vi "Read Pinch Strenght.vi"(6 "Multi-pinch":bool, 8 "Error In":errorcluster, 11 "Leap Handle In":T1) -> (0 "Error Out":errorcluster, 1 "Finger pinch":bool[](array[boolean]), 2 "Pinch Strength":sgl, 3 "Leap Handle Out":T1)   [LabVIEW 2014]
doc: "<b>Leap Read</b> requests and parses a <b>Frame</b> of data from the Leap Motion Controller. All the data associated with the Frame is organized into a LabVIEW cluster for accessibility.\n\nSpecifics about the data in the Frame cluster can be found by going to <b>Help » Leap Motion Controller Help</b> inside of LabVIEW"
uses:
  Typedef 2.0/Leap Handle.ctl
  C:/Users/Arquilla/Desktop/Smart Wristband/Leap Motion VIs 2.0/LeapCSharp.NET4.0.dll
  LeapCSharp.NET4.0.dll
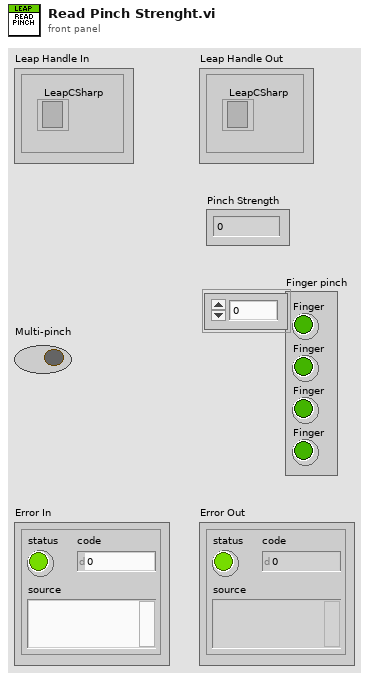
[diagram p1: front panel]
types:
  T1 = typedef "Leap Handle.ctl" = cluster{"LeapCSharp":refnum<k24>}
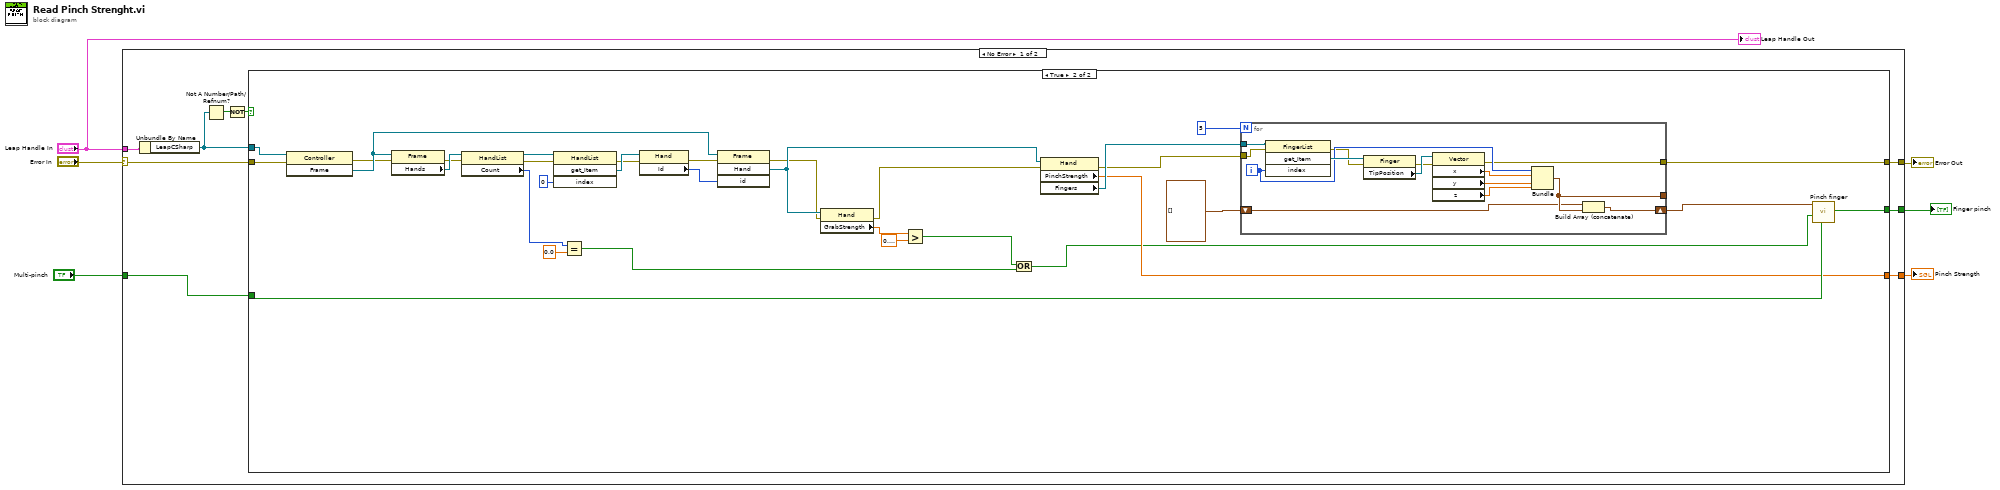
[diagram p0: block diagram]
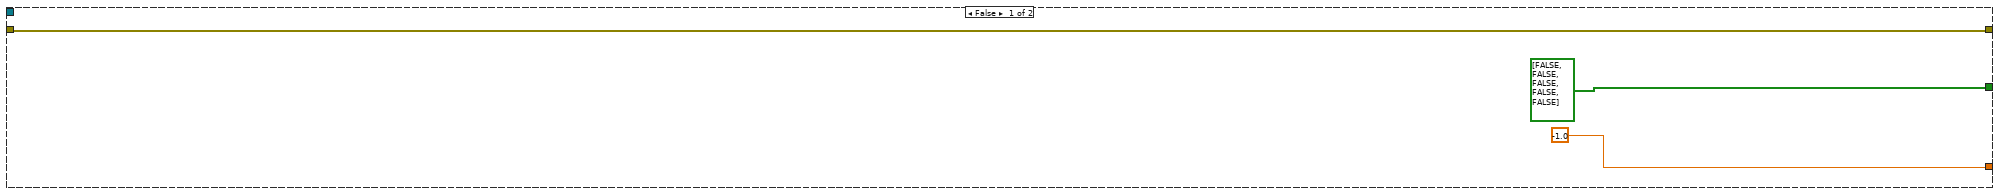
[diagram p2: hidden frame]
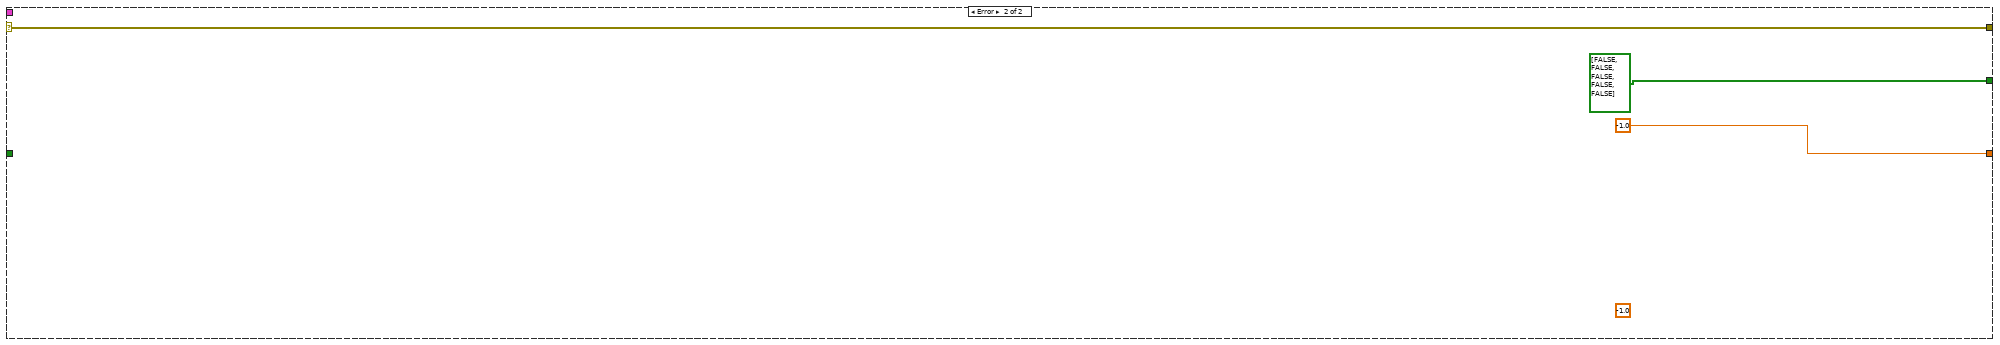
[diagram p3: hidden frame]
diagram:
  n1 = case shown="No Error" "Error In" {
    selector: "Error In" -> [w14 w67]
    tunnel: "Leap Handle In" -> [w15 _]
    tunnel: [w13 w67] -> w5
    tunnel: [w9 sgl -1.0 ("PinchStrength")] -> w3
    tunnel: [w8 bool[] [FALSE, FALSE, FALSE, FALSE, FALSE] ("Finger pinch")] -> w2
    tunnel: "Multi-pinch" -> [w7 _]
    frame No Error {
      n2 = Unbundle By Name(w15) -> ("LeapCSharp"=w10:refnum<k24>)
      n3 = Not A Number/Path/Refnum?(number/path/refnum=w10) -> (NaN/Path/Refnum?=w12:bool)
      n4 = Not(x=w12) -> (.not. x?=w11:bool)
      n5 = case shown="True" w11 {
        tunnel: w14 -> [w18 w38]
        tunnel: [w18 w36] -> w13
        tunnel: w10 -> [_ w39]
        tunnel: [sgl -1.0 ("GrabStrength") w24] -> w9
        tunnel: [bool[] [FALSE, FALSE, FALSE, FALSE, FALSE] ("Finger pinch") w37] -> w8
        tunnel: w7 -> [_ w35]
        frame False {
        }
        frame True {
          n6 = invoke class="Controller" method="Frame"(reference=w39, error in=w38) -> (error out=w44:errorcluster, "Frame"=w45:refnum<k24>)  [unwired: 1 in, 1 out]
          n7 = property class="Frame"(reference=w45, error in=w44) -> (error out=w43:errorcluster, "Hands"=w50:refnum<k24>)  [unwired: 1 out]
          n8 = property class="HandList"(reference=w50, error in=w43) -> (reference out=w49:refnum<k24>, error out=w42:errorcluster, "Count"=w22:i32)
          n9 = invoke class="HandList" method="get_Item"(reference=w49, error in=w42, "index"=0) -> (error out=w41:errorcluster, "get_Item"=w47:refnum<k24>)  [unwired: 1 in, 2 out]
          n10 = Equal?(x=w22, y=0.0) -> (x = y?=w20:bool)
          n11 = property class="Hand"(reference=w47, error in=w41) -> (error out=w40:errorcluster, "Id"=w46:i32)  [unwired: 1 out]
          n12 = invoke class="Frame" method="Hand"(reference=w45, error in=w40, "id"=w46) -> (error out=w27:errorcluster, "Hand"=w29:refnum<k24>)  [unwired: 1 in, 2 out]
          n13 = property class="Hand"(reference=w29, error in=w27) -> (error out=w26:errorcluster, "GrabStrength"=w28:sgl)  [unwired: 1 out]
          n14 = Greater?(x=w28, y=sgl 0.2) -> (0:w21:bool)
          n15 = Or(x=w21, y=w20) -> (x .or. y?=w19:bool)
          n16 = property class="Hand"(reference=w29, error in=w26) -> (error out=w30:errorcluster, "PinchStrength"=w24:sgl, "Fingers"=w33:refnum<k24>)  [unwired: 1 out]
          n17 = for {
            N: 5 -> [_]
            tunnel: w33 -> [w64]
            tunnel: [w57] -> _
            shift-right: [w56] -> w31
            shift-left: cluster{i32, "x":sgl, "y":sgl, "z":sgl}[] [] -> [w55]
            tunnel: w30 -> [w54]
            tunnel: [w51] -> w36
            i -> [w58]
            n18 = invoke class="FingerList" method="get_Item"(reference=w64, error in=w54, "index"=w58) -> (error out=w53:errorcluster, "get_Item"=w63:refnum<k24>)  [unwired: 1 in, 2 out]
            n19 = property class="Finger"(reference=w63, error in=w53) -> (error out=w52:errorcluster, "TipPosition"=w62:refnum<k24>)  [unwired: 1 out]
            n20 = property class="Vector"(reference=w62, error in=w52) -> (error out=w51:errorcluster, "x"=w61:sgl, "y"=w60:sgl, "z"=w59:sgl)  [unwired: 1 out]
            n21 = Bundle(w58, "x"=w61, "y"=w60, "z"=w59) -> (w57:cluster{i32, "x":sgl, "y":sgl, "z":sgl})  [unwired: 1 in]
            n22 = Build Array (concatenate)(w55, w57) -> (w56:cluster{i32, "x":sgl, "y":sgl, "z":sgl}[])
          }
          n23 = call "Pinch finger.vi"("Multi-pinch enabled"=w35, "Boolean"=w19, "Finger Vector In"=w31) -> ("Finger pinch"=w37:bool[])  [unwired: 8 in]
        }
      }
    }
    frame Error {
      (unwired) sgl -1.0 ("Dot")
    }
  }
  "Error Out" <- w5
  "Pinch Strength" <- w3
  "Finger pinch" <- w2
  "Leap Handle Out" <- "Leap Handle In"
